vi "HP8753 Set Sweep REFERENCE.vi"(0 "VISA session":refnum<visa-resource-name>, 1 "sweep type (0 : linear)":u16(ring) items=["linear sweep", "logarithmic sweep", "frequency list", "CW time sweep", "power sweep"], 2 "start/center":dbl=1000000000.0 format="%.2e", 3 "start/center units (1 : Hz/dBm)":u16(ring) items=["Hz / dBm", "kHz / dBm", "MHz / dBm", "GHz / dBm"], 5 "CW freq (Hz)":dbl=1000.0 format="%.2e", 6 "frequency list":T1(array[cluster]) {"num points" min=1 max=1632; "step (Hz)" format="%.2e"; "stop (Hz)" format="%.2e"; "start (Hz)" format="%.2e"}, 7 "num points":u16(ring)=5 items=["3", "11", "21 ('20) / 26 ('53)", "51", "101", "201", "401", "801", "1601"], 9 "sweep time (sec)":dbl=0.1 format="%.2f", 11 "error in (no error)":errorcluster, 12 "t: start/stop  f: center/span":bool=TRUE, 13 "stop/span":dbl=10000000000.0 format="%.2e", 14 "stop/span units (1 : Hz/dBm)":u16(ring) items=["Hz / dBm", "kHz / dBm", "MHz / dBm", "GHz / dBm"]) -> (4 "dup VISA session":refnum<visa-resource-name>, 15 "error out":errorcluster)   [LabVIEW 2011]
doc: "This VI sets up sweeps for the HP8753B Network Analyzer. The sweep type is set with the \"sweep type\" text ring. The functions of the other controls are determined by the \"sweep type\" setting."
panel:
  # "power sweeps and CW time sweeps"
  # "all sweeps except freq list sweeps"
  # "all sweeps especially CW time sweeps"
  # "linear and log sweeps and power sweeps"
  # "frequency list sweeps"
  # "start/stop"
  # "center/span"
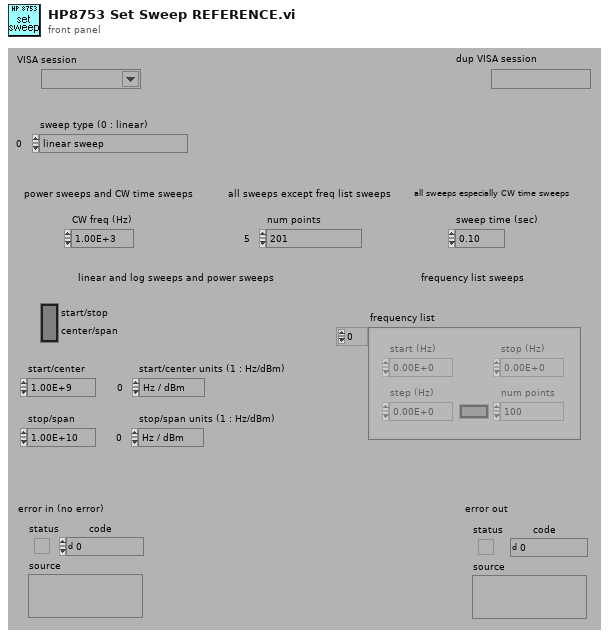
[diagram p1: front panel]
types:
  T1 = cluster{"start (Hz)":dbl, "stop (Hz)":dbl, bool, "step (Hz)":dbl, "num points":u16}[]
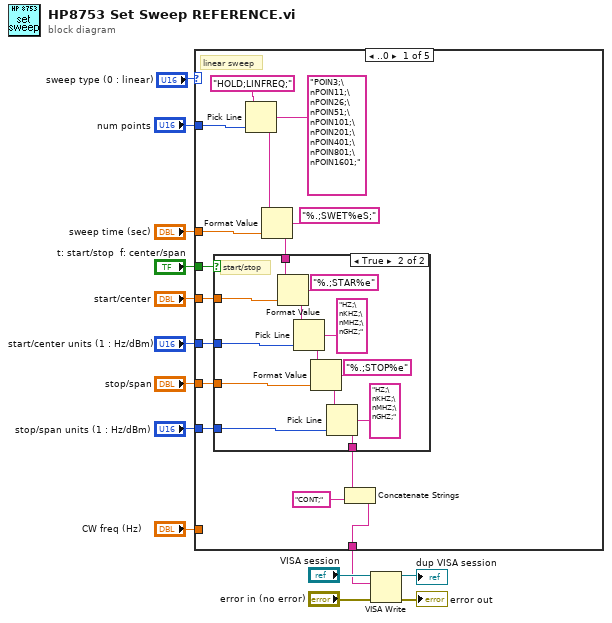
[diagram p0: block diagram]
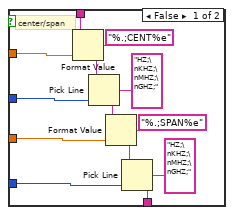
[diagram p2: hidden frame]
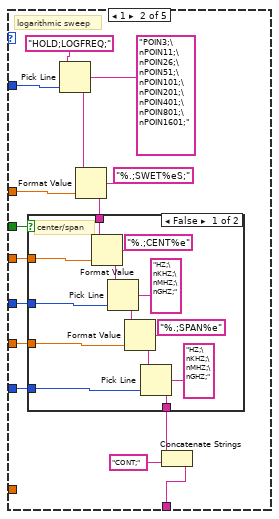
[diagram p3: hidden frame]
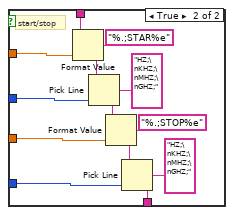
[diagram p4: hidden frame]
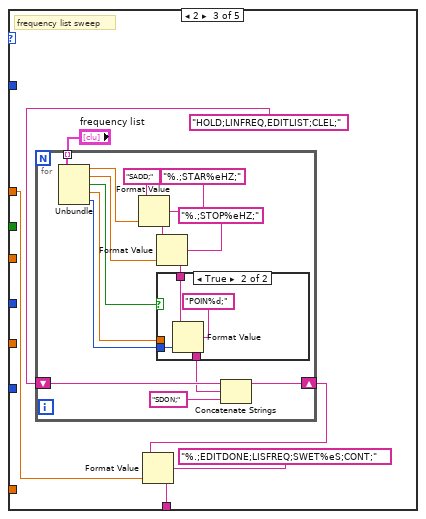
[diagram p5: hidden frame]
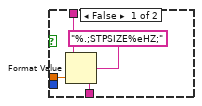
[diagram p6: hidden frame]
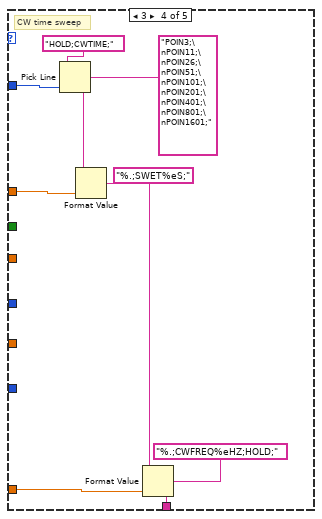
[diagram p7: hidden frame]
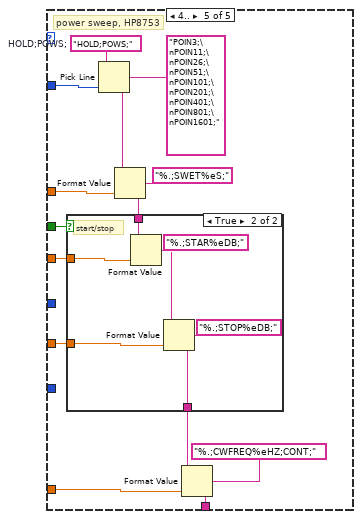
[diagram p8: hidden frame]
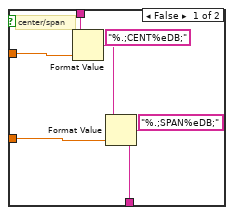
[diagram p9: hidden frame]
diagram:
  n1 = case shown="..0" "sweep type (0 : linear)" {
    tunnel: "num points" -> [w27 w68 _ w133 w147]
    tunnel: "sweep time (sec)" -> [w24 w65 w100 w130 w144]
    tunnel: "t: start/stop  f: center/span" -> [w23 w64 _ _ w143]
    tunnel: "start/center" -> [w21 w62 _ _ w141]
    tunnel: "start/center units (1 : Hz/dBm)" -> [w20 w61 _ _ _]
    tunnel: "stop/span" -> [w19 w60 _ _ w140]
    tunnel: "stop/span units (1 : Hz/dBm)" -> [w18 w59 _ _ _]
    tunnel: "CW freq (Hz)" -> [_ _ _ w128 w136]
    tunnel: [w15 w56 w98 w126 w137] -> w1
    frame ..0 {
      # "linear sweep"
      n2 = Pick Line(string ("")="HOLD;LINFREQ;", multi-line string="POIN3;\nPOIN11;\nPOIN26;\nPOIN51;\nPOIN101;\nPOIN201;\nPOIN401;\nPOIN801;\nPOIN1601;", line index=w27) -> (output string=w26:string)
      n3 = Format Value(string ("")=w26, format string="%.;SWET%eS;", value (0)=w24) -> (output string=w22:string)
      n4 = case shown="True" w23 {
        tunnel: w22 -> [w42 w55]
        tunnel: w21 -> [w41 w54]
        tunnel: w20 -> [w37 w50]
        tunnel: w19 -> [w32 w45]
        tunnel: w18 -> [w31 w44]
        tunnel: [w30 w43] -> w16
        frame False {
          # "center/span"
          n5 = Format Value(string ("")=w42, format string="%.;CENT%e", value (0)=w41) -> (output string=w39:string)
          n6 = Pick Line(string ("")=w39, multi-line string="HZ;\nKHZ;\nMHZ;\nGHZ;", line index=w37) -> (output string=w33:string)
          n7 = Format Value(string ("")=w33, format string="%.;SPAN%e", value (0)=w32) -> (output string=w35:string)
          n8 = Pick Line(string ("")=w35, multi-line string="HZ;\nKHZ;\nMHZ;\nGHZ;", line index=w31) -> (output string=w30:string)
        }
        frame True {
          # "start/stop"
          n9 = Format Value(string ("")=w55, format string="%.;STAR%e", value (0)=w54) -> (output string=w52:string)
          n10 = Pick Line(string ("")=w52, multi-line string="HZ;\nKHZ;\nMHZ;\nGHZ;", line index=w50) -> (output string=w46:string)
          n11 = Format Value(string ("")=w46, format string="%.;STOP%e", value (0)=w45) -> (output string=w48:string)
          n12 = Pick Line(string ("")=w48, multi-line string="HZ;\nKHZ;\nMHZ;\nGHZ;", line index=w44) -> (output string=w43:string)
        }
      }
      n13 = Concatenate Strings(w16, "CONT;") -> (w15:string)
    }
    frame 1 {
      # "logarithmic sweep"
      n14 = Pick Line(string ("")="HOLD;LOGFREQ;", multi-line string="POIN3;\nPOIN11;\nPOIN26;\nPOIN51;\nPOIN101;\nPOIN201;\nPOIN401;\nPOIN801;\nPOIN1601;", line index=w68) -> (output string=w67:string)
      n15 = Format Value(string ("")=w67, format string="%.;SWET%eS;", value (0)=w65) -> (output string=w63:string)
      n16 = case shown="False" w64 {
        tunnel: w63 -> [w83 w96]
        tunnel: w62 -> [w82 w95]
        tunnel: w61 -> [w78 w91]
        tunnel: w60 -> [w73 w86]
        tunnel: w59 -> [w72 w85]
        tunnel: [w71 w84] -> w57
        frame False {
          # "center/span"
          n17 = Format Value(string ("")=w83, format string="%.;CENT%e", value (0)=w82) -> (output string=w80:string)
          n18 = Pick Line(string ("")=w80, multi-line string="HZ;\nKHZ;\nMHZ;\nGHZ;", line index=w78) -> (output string=w74:string)
          n19 = Format Value(string ("")=w74, format string="%.;SPAN%e", value (0)=w73) -> (output string=w76:string)
          n20 = Pick Line(string ("")=w76, multi-line string="HZ;\nKHZ;\nMHZ;\nGHZ;", line index=w72) -> (output string=w71:string)
        }
        frame True {
          # "start/stop"
          n21 = Format Value(string ("")=w96, format string="%.;STAR%e", value (0)=w95) -> (output string=w93:string)
          n22 = Pick Line(string ("")=w93, multi-line string="HZ;\nKHZ;\nMHZ;\nGHZ;", line index=w91) -> (output string=w87:string)
          n23 = Format Value(string ("")=w87, format string="%.;STOP%e", value (0)=w86) -> (output string=w89:string)
          n24 = Pick Line(string ("")=w89, multi-line string="HZ;\nKHZ;\nMHZ;\nGHZ;", line index=w85) -> (output string=w84:string)
        }
      }
      n25 = Concatenate Strings(w57, "CONT;") -> (w56:string)
    }
    frame 2 {
      # "frequency list sweep"
      n26 = for {
        tunnel: "frequency list" -> [w117] mode=indexing
        shift-right: [w105] -> w99
        shift-left: "HOLD;LINFREQ,EDITLIST;CLEL;" -> [w108]
        n27 = Unbundle(w117) -> ("start (Hz)"=w103:dbl, "stop (Hz)"=w104:dbl, w112:bool, "step (Hz)"=w110:dbl, "num points"=w109:u16)
        n28 = Format Value(string ("")="SADD;", format string="%.;STAR%eHZ;", value (0)=w103) -> (output string=w113:string)
        n29 = Format Value(string ("")=w113, format string="%.;STOP%eHZ;", value (0)=w104) -> (output string=w111:string)
        n30 = case shown="True" w112 {
          tunnel: w111 -> [w120 w124]
          tunnel: w110 -> [w119 _]
          tunnel: w109 -> [_ w123]
          tunnel: [w118 w122] -> w107
          frame False {
            n31 = Format Value(string ("")=w120, format string="%.;STPSIZE%eHZ;", value (0)=w119) -> (output string=w118:string)
          }
          frame True {
            n32 = Format Value(string ("")=w124, format string="POIN%d;", value (0)=w123) -> (output string=w122:string)
          }
        }
        n33 = Concatenate Strings(w108, w107, "SDON;") -> (w105:string)
      }
      n34 = Format Value(string ("")=w99, format string="%.;EDITDONE;LISFREQ;SWET%eS;CONT;", value (0)=w100) -> (output string=w98:string)
    }
    frame 3 {
      # "CW time sweep"
      n35 = Pick Line(string ("")="HOLD;CWTIME;", multi-line string="POIN3;\nPOIN11;\nPOIN26;\nPOIN51;\nPOIN101;\nPOIN201;\nPOIN401;\nPOIN801;\nPOIN1601;", line index=w133) -> (output string=w132:string)
      n36 = Format Value(string ("")=w132, format string="%.;SWET%eS;", value (0)=w130) -> (output string=w129:string)
      n37 = Format Value(string ("")=w129, format string="%.;CWFREQ%eHZ;HOLD;", value (0)=w128) -> (output string=w126:string)
    }
    frame 4.. {
      w149 = "HOLD;POWS;"  # HOLD;POWS;
      # "power sweep, HP8753"
      n38 = Pick Line(string ("")=w149, multi-line string="POIN3;\nPOIN11;\nPOIN26;\nPOIN51;\nPOIN101;\nPOIN201;\nPOIN401;\nPOIN801;\nPOIN1601;", line index=w147) -> (output string=w146:string)
      n39 = Format Value(string ("")=w146, format string="%.;SWET%eS;", value (0)=w144) -> (output string=w142:string)
      n40 = case shown="True" w143 {
        tunnel: w142 -> [w156 w163]
        tunnel: w141 -> [w155 w162]
        tunnel: w140 -> [w152 w158]
        tunnel: [w150 w157] -> w138
        frame False {
          # "center/span"
          n41 = Format Value(string ("")=w156, format string="%.;CENT%eDB;", value (0)=w155) -> (output string=w151:string)
          n42 = Format Value(string ("")=w151, format string="%.;SPAN%eDB;", value (0)=w152) -> (output string=w150:string)
        }
        frame True {
          # "start/stop"
          n43 = Format Value(string ("")=w163, format string="%.;STAR%eDB;", value (0)=w162) -> (output string=w160:string)
          n44 = Format Value(string ("")=w160, format string="%.;STOP%eDB;", value (0)=w158) -> (output string=w157:string)
        }
      }
      n45 = Format Value(string ("")=w138, format string="%.;CWFREQ%eHZ;CONT;", value (0)=w136) -> (output string=w137:string)
    }
  }
  n46 = VISA Write(VISA resource name="VISA session", write buffer=w1, error in (no error)="error in (no error)") -> (VISA resource name out=→"dup VISA session":refnum<visa-resource-name>, error out=→"error out":errorcluster)  [unwired: 1 out]
